vi "HostCameraRemoteControl.vi"() -> ()   [LabVIEW 2024]
panel:
  out "stream overhead":u32
  out "byte_pending":i32
  out "error out":errorcluster
  out "frame idx":string
  in  "OK Button":bool
  out "Img":dbl[][](graph)
  in  "stop":bool
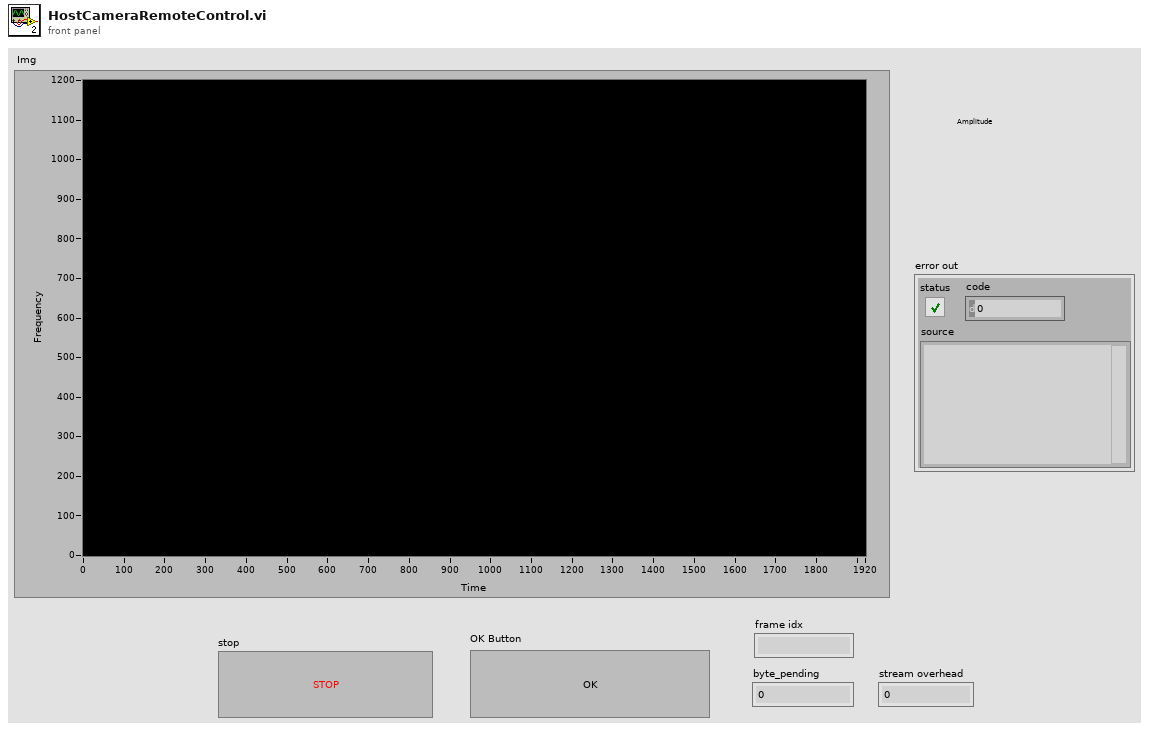
[diagram p1: front panel]
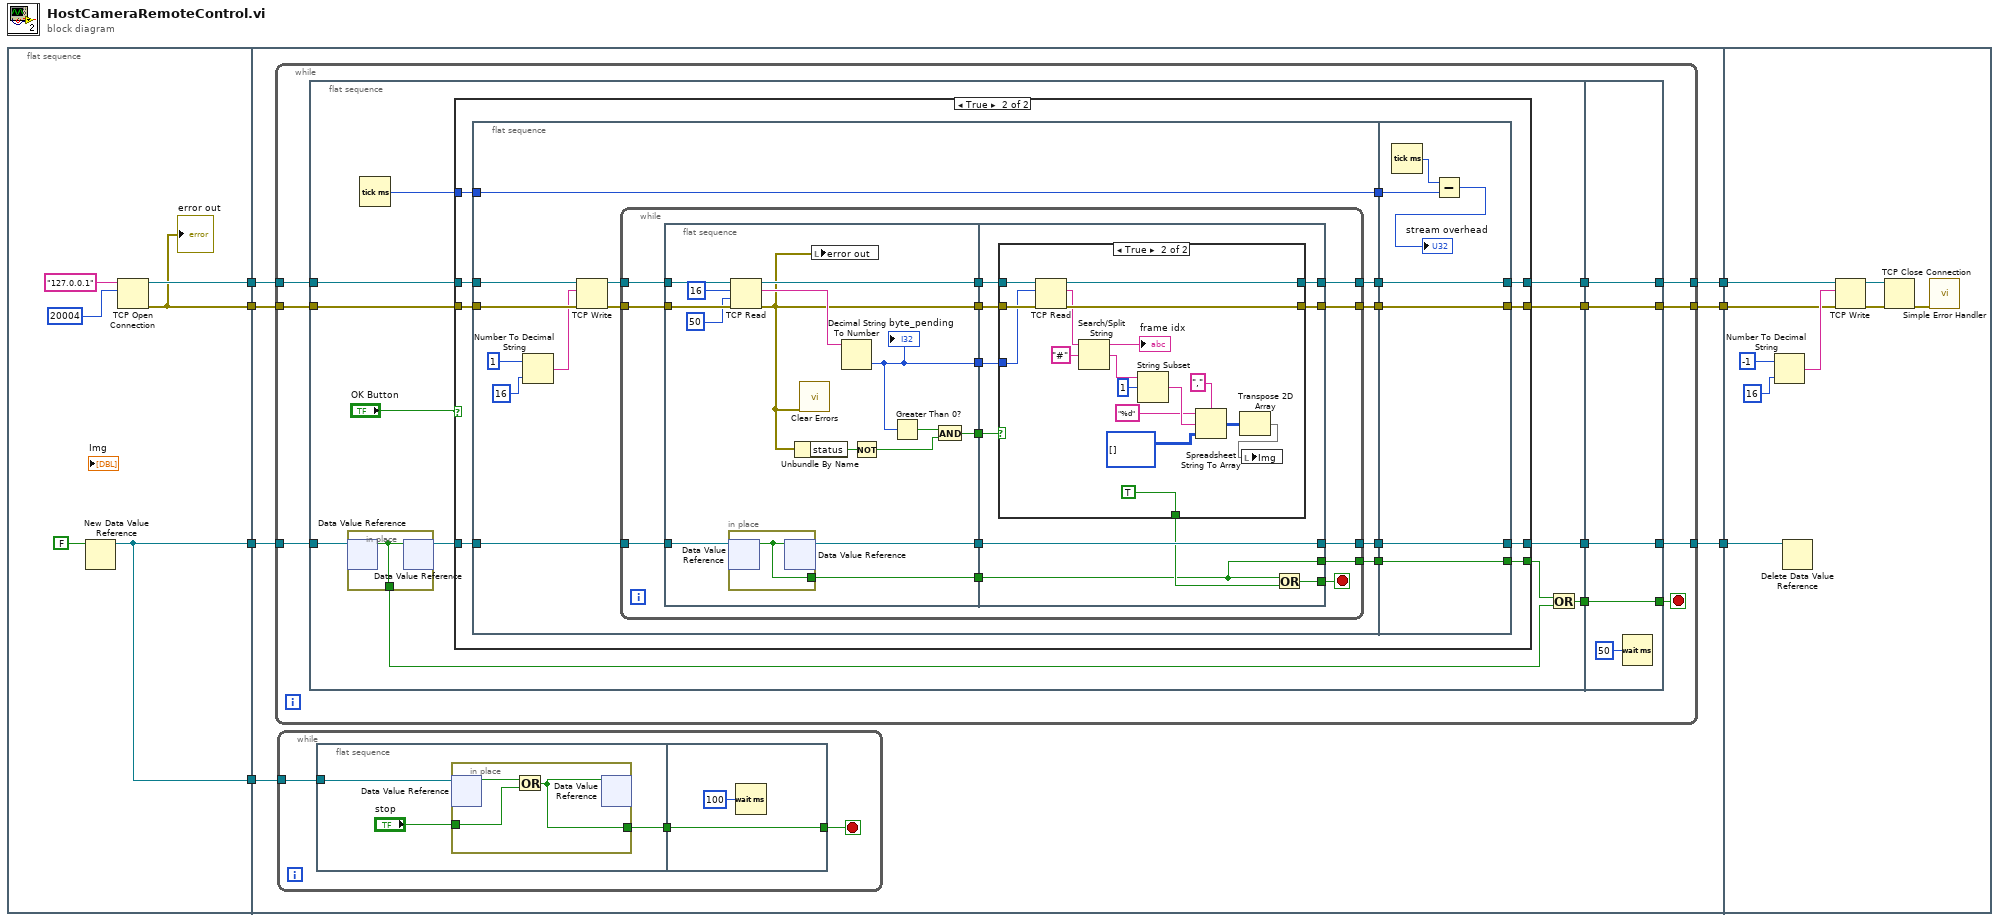
[diagram p0: block diagram]
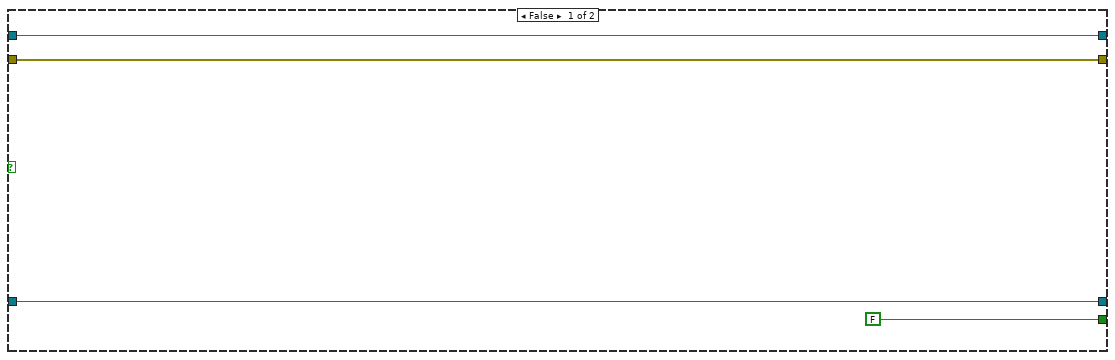
[diagram p2: hidden frame]
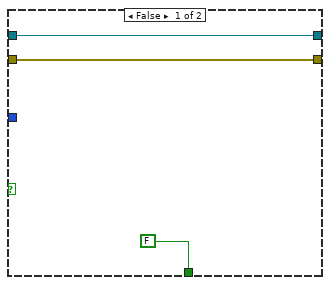
[diagram p3: hidden frame]
diagram:
  n1 = flat-sequence {
    tunnel: [w12] -> w7
    tunnel: [w9] -> w6
    tunnel: [w10] -> w5
    tunnel: [w10] -> w4
    tunnel: w7 -> [w20]
    tunnel: w6 -> [w19]
    tunnel: w5 -> [w18]
    tunnel: w4 -> [w17]
    tunnel: [w16] -> w3
    tunnel: [w15] -> w2
    tunnel: [w14] -> w1
    tunnel: w3 -> [w158]
    tunnel: w2 -> [w163]
    tunnel: w1 -> [w162]
    frame #0 {
      n2 = New Data Value Reference(data value=FALSE) -> (data value reference=w10:refnum<data-value>)  [unwired: 1 in, 1 out]
      n3 = TCP Open Connection(address="127.0.0.1", remote port or service name=20004) -> (connection ID=w12:refnum<k5>, error out=w9:errorcluster)  [unwired: 3 in]
      "error out" <- w9
    }
    frame #1 {
      n4 = while {
        tunnel: w20 -> [w42]
        tunnel: w19 -> [w41]
        tunnel: w18 -> [w40]
        tunnel: [w39] -> w16
        tunnel: [w38] -> w15
        tunnel: [w37] -> w14
        stop <- w36 stop-if-true
        n5 = flat-sequence {
          tunnel: w40 -> [w52]
          tunnel: w41 -> [w53]
          tunnel: w42 -> [w54]
          tunnel: [w50] -> w35
          tunnel: [w49] -> w34
          tunnel: [w48] -> w33
          tunnel: [w45] -> w32
          tunnel: [w154] -> w36
          tunnel: [w155] -> w37
          tunnel: [w156] -> w38
          tunnel: [w157] -> w39
          tunnel: w35 -> [w157]
          tunnel: w34 -> [w156]
          tunnel: w33 -> [w155]
          tunnel: w32 -> [w154]
          frame #0 {
            n6 = in-place {
              in-place-border: [w152] -> w46
              n7 = in-place-dvr #1(w52) -> (w152:bool)  [unwired: 1 out]
              n8 = in-place-dvr #1(w152) -> (w51:refnum<data-value>)  [unwired: 1 out]
            }
            n9 = Tick Count (ms)() -> (millisecond timer value=w43:u32)
            n10 = case shown="True" "OK Button" {
              tunnel: w54 -> [w58 w71]
              tunnel: w53 -> [w57 w70]
              tunnel: w51 -> [w56 w69]
              tunnel: [w56 w68] -> w50
              tunnel: [w58 w67] -> w49
              tunnel: [w57 w66] -> w48
              tunnel: [FALSE w65] -> w47
              tunnel: w43 -> [_ w60]
              frame False {
              }
              frame True {
                n11 = flat-sequence {
                  tunnel: w71 -> [w84]
                  tunnel: w70 -> [w83]
                  tunnel: w69 -> [w80]
                  tunnel: [w79] -> w64
                  tunnel: [w78] -> w63
                  tunnel: [w77] -> w62
                  tunnel: [w76] -> w61
                  tunnel: w60 -> [w72]
                  tunnel: [w72] -> w59
                  tunnel: [w148] -> w65
                  tunnel: [w149] -> w66
                  tunnel: [w150] -> w67
                  tunnel: [w151] -> w68
                  tunnel: w64 -> [w151]
                  tunnel: w63 -> [w150]
                  tunnel: w62 -> [w149]
                  tunnel: w61 -> [w148]
                  tunnel: w59 -> [w146]
                  frame #0 {
                    n12 = Number To Decimal String(number=1, width (-)=i16 16) -> (decimal integer string=w74:string)
                    n13 = TCP Write(connection ID=w84, data in=w74, error in (no error)=w83) -> (connection ID out=w82:refnum<k5>, error out=w81:errorcluster)  [unwired: 1 in, 1 out]
                    n14 = while {
                      tunnel: w82 -> [w98]
                      tunnel: w81 -> [w97]
                      tunnel: w80 -> [w94]
                      tunnel: [w89] -> w79
                      tunnel: [w88] -> w78
                      tunnel: [w87] -> w77
                      tunnel: [w85] -> w76
                      stop <- w86 stop-if-true
                      n15 = flat-sequence {
                        tunnel: w98 -> [w113]
                        tunnel: w97 -> [w112]
                        tunnel: [w109] -> w96
                        tunnel: [w100] -> w95
                        tunnel: w94 -> [w108]
                        tunnel: [w107] -> w93
                        tunnel: [w99] -> w92
                        tunnel: [w102] -> w91
                        tunnel: [w101] -> w90
                        tunnel: w96 -> [w124]
                        tunnel: w95 -> [w123]
                        tunnel: w93 -> [w118]
                        tunnel: w92 -> [w122]
                        tunnel: w91 -> [w121]
                        tunnel: [w120] -> w88
                        tunnel: [w119] -> w87
                        tunnel: w90 -> [w116]
                        tunnel: [w118] -> w89
                        tunnel: [w115] -> w86
                        tunnel: [w116] -> w85
                        frame #0 {
                          n16 = in-place {
                            in-place-border: [w114] -> w101
                            n17 = in-place-dvr #2(w108) -> (w114:bool)  [unwired: 1 out]
                            n18 = in-place-dvr #2(w114) -> (w107:refnum<data-value>)  [unwired: 1 out]
                          }
                          n19 = TCP Read(connection ID=w113, bytes to read=16, error in (no error)=w112, 9:50 ("timeout ms (25000)")) -> (connection ID out=w109:refnum<k5>, data out=w106:string, error out=w100:errorcluster)  [unwired: 1 in]
                          n20 = Unbundle By Name(w100) -> ("status"=w105:bool)
                          n21 = call <vilib>:"Clear Errors.vi"("error in (no error)"=w100) -> ()  [unwired: 5 in, 2 out]
                          n22 = local write "error out"(w100) -> ()
                          n23 = Decimal String To Number(string=w106) -> (number=w99:i32)  [unwired: 2 in, 1 out]
                          "byte_pending" <- w99
                          n24 = Not(x=w105) -> (.not. x?=w103:bool)
                          n25 = Greater Than 0?(x=w99) -> (x > 0?=w104:bool)
                          n26 = And(x=w104, y=w103) -> (x .and. y?=w102:bool)
                        }
                        frame #1 {
                          n27 = case shown="True" w121 {
                            tunnel: w124 -> [w127 w144]
                            tunnel: w123 -> [w126 w143]
                            tunnel: w122 -> [_ w142]
                            tunnel: [w127 w141] -> w120
                            tunnel: [w126 w140] -> w119
                            tunnel: [FALSE TRUE] -> w117
                            frame False {
                            }
                            frame True {
                              n28 = TCP Read(connection ID=w144, bytes to read=w142, error in (no error)=w143) -> (connection ID out=w141:refnum<k5>, data out=w138:string, error out=w140:errorcluster)  [unwired: 2 in]
                              n29 = Search/Split String(string=w138, search string/char (-)="#") -> (substring before match=→"frame idx":string, match + rest of string=w136:string)  [unwired: 1 in, 1 out]
                              n30 = String Subset(string=w136, offset (0)=1) -> (substring=w134:string)  [unwired: 1 in]
                              n31 = Spreadsheet String To Array(delimiter (Tab)=",", format string="%d", spreadsheet string=w134, array type (2D Dbl)=i32[][] []) -> (array=w130:i32[][])
                              n32 = Transpose 2D Array(2D array=w130) -> (transposed array=w129:i32[][])
                              n33 = local write "Img"(w129) -> ()
                            }
                          }
                          n34 = Or(x=w116, y=w117) -> (x .or. y?=w115:bool)
                        }
                      }
                    }
                  }
                  frame #1 {
                    n35 = Tick Count (ms)() -> (millisecond timer value=w147:u32)
                    n36 = Subtract(x=w147, y=w146) -> (x-y=→"stream overhead":u32)
                  }
                }
              }
            }
            n37 = Or(x=w47, y=w46) -> (x .or. y?=w45:bool)
          }
          frame #1 {
            n38 = Wait (ms)(milliseconds to wait=u32 50) -> ()  [unwired: 1 out]
          }
        }
      }
      n39 = while {
        tunnel: w17 -> [w23]
        stop <- w21 stop-if-true
        n40 = flat-sequence {
          tunnel: w23 -> [w26]
          tunnel: [w24] -> w22
          tunnel: w22 -> [w31]
          tunnel: [w31] -> w21
          frame #0 {
            n41 = in-place {
              in-place-border: "stop" -> [w28]
              in-place-border: [w27] -> w24
              n42 = in-place-dvr #3(w26) -> (w29:bool)  [unwired: 1 out]
              n43 = Or(x=w29, y=w28) -> (x .or. y?=w27:bool)
              n44 = in-place-dvr #3(w27) -> ()  [unwired: 2 out]
            }
          }
          frame #1 {
            n45 = Wait (ms)(milliseconds to wait=u32 100) -> ()  [unwired: 1 out]
          }
        }
      }
    }
    frame #2 {
      n46 = Number To Decimal String(number=-1, width (-)=i16 16) -> (decimal integer string=w165:string)
      n47 = Delete Data Value Reference(data value reference=w158) -> ()  [unwired: 1 in, 2 out]
      n48 = TCP Write(connection ID=w163, data in=w165, error in (no error)=w162) -> (connection ID out=w161:refnum<k5>, error out=w160:errorcluster)  [unwired: 1 in, 1 out]
      n49 = TCP Close Connection(connection ID=w161, error in (no error)=w160) -> (error out=w159:errorcluster)  [unwired: 1 in, 1 out]
      n50 = call <vilib>:"Simple Error Handler.vi"("error in (no error)"=w159) -> ()  [unwired: 4 in, 5 out]
    }
  }
